vi "find_bright_column.vi"(7 "Right border":i32, 9 "Left border":i32, 10 "filter size":i32=10, 11 "Image":T1) -> (3 "peak column":i32)   [LabVIEW 2016]
uses:
  <vilib>/vision/Image Controls.llb/IMAQ Image.ctl
  <vilib>/Analysis/baseanly.llb/Mean (DBL).vi
  <vilib>/Analysis/NI_AALBase.lvlib
  <vilib>/vision/NI_Vision_Development_Module.lvlib
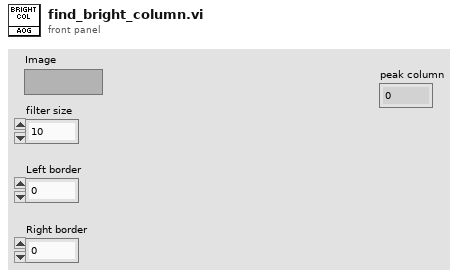
[diagram p1: front panel]
types:
  T1 = typedef "IMAQ Image.ctl" = refnum<image>
  T2 = typedef "Image Type" = u32
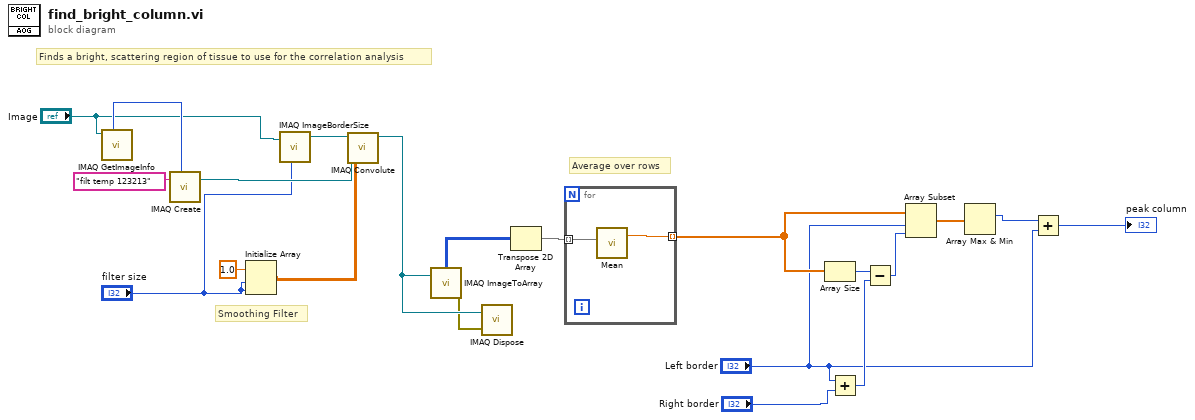
[diagram p0: block diagram]
diagram:
  # "Average over rows"
  # "Smoothing Filter"
  # "Finds a bright, scattering region of tissue to use for the correlation analysis"
  n1 = call "IMAQ GetImageInfo"("Image"="Image") -> ("Image Type"=w5:T2)  [unwired: 3 in, 7 out]
  n2 = call "IMAQ Create"("Image Name"="filt temp 123213", "Image Type"=w5) -> ("New Image"=w18:T1)  [unwired: 3 in, 1 out]
  n3 = Initialize Array(1.0 ("element"), "filter size", "filter size") -> (w14:dbl[][])
  n4 = call "IMAQ ImageBorderSize"("Image"="Image", "Image border size in"="filter size") -> ("Image Out"=w8:T1)  [unwired: 2 in, 2 out]
  n5 = call "IMAQ Convolute"("Kernel"=w14, "Image Dst"=w18, "Image Src"=w8) -> ("Image Dst Out"=w17:T1)  [unwired: 7 in, 1 out]
  n6 = call "IMAQ ImageToArray"("Image"=w17) -> ("error out"=w16:errorcluster, "Image Pixels (U8)"=w21:u8[][])  [unwired: 3 in, 3 out]
  n7 = call "IMAQ Dispose"("Image"=w17, "error in (no error)"=w16) -> ()  [unwired: 4 in, 1 out]
  n8 = Transpose 2D Array(2D array=w21) -> (transposed array=w20:u8[][])
  n9 = for {
    tunnel: w20 -> [w23] mode=indexing
    tunnel: [w22] -> w12 mode=indexing
    n10 = call-poly <vilib>:"Mean.vi"("X"=w23) -> ("mean"=w22:dbl)  [unwired: 1 out]
  }
  n11 = Array Size(array=w12) -> (size(s)=w10:i32)
  n12 = Add(x="Left border", y="Right border") -> (x+y=w6:i32)
  n13 = Subtract(x=w10, y=w6) -> (x-y=w9:i32)
  n14 = Array Subset(array=w12, index="Left border", length=w9) -> (w11:dbl[])
  n15 = Array Max & Min(array=w11) -> (max index (indices)=w3:i32)  [unwired: 3 out]
  n16 = Add(x=w3, y="Left border") -> (x+y=→"peak column":i32)
